vi "Script Rich to Flat Oneof Conversion.vi"(5 "element metadata":T1={"Field Name"="", "Embedded Message Name"="", "Protobuf Index"=1, "MessageElementType"=enum."StringValue", "Repeated"=FALSE, "Is in Oneof"=FALSE, "Oneof Container Name"=""}, 7 "library in":refnum<vi>, 8 "error in (no error)":errorcluster, 9 "unbundler":refnum<vi>, 10 "bundler":refnum<vi>, 11 "vi in":refnum<vi>) -> (0 "error out":errorcluster, 3 "vi out":refnum<vi>)   [LabVIEW 2019, in "gRPC Template Creation Utility.lvlib"]
uses:
  gRPC Template Creation Utility.lvlib
  OneOf Constants/OneOfConstantsEnum.ctl
  TypeDefs/Message Element Type.ctl
  TypeDefs/Message Element Metadata (Scripting).ctl
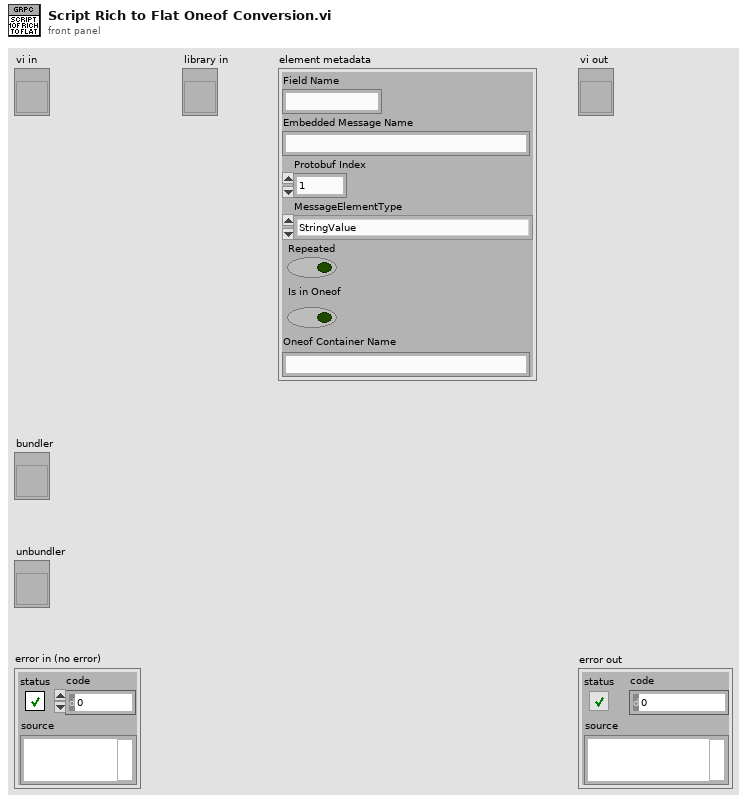
[diagram p1: front panel]
types:
  T1 = typedef "gRPC Template Creation Utility.lvlib/Message Element Metadata (Scripting).ctl" = cluster{"Field Name":string, "Embedded Message Name":string, "Protobuf Index":i32, "MessageElementType":T2, "Repeated":bool, "Is in Oneof":bool, "Oneof Container Name":string}
  T2 = typedef "gRPC Template Creation Utility.lvlib/Message Element Type.ctl" = enum32{"Int32Value", "FloatValue", "DoubleValue", "BoolValue", "StringValue", "MessageValue", "Int64Value", "UInt32Value", "UInt64Value", "EnumValue", "Bytes", "Fixed64", "Fixed32", "SFixed64", "SFixed32", "SInt64", "SInt32"}
  T3 = typedef "gRPC Template Creation Utility.lvlib/OneOfConstantsEnum.ctl" = enum16{"FlatToRichVIPrefix", "RichToFlatVIPrefix", "FlatTypeDefSuffix"}
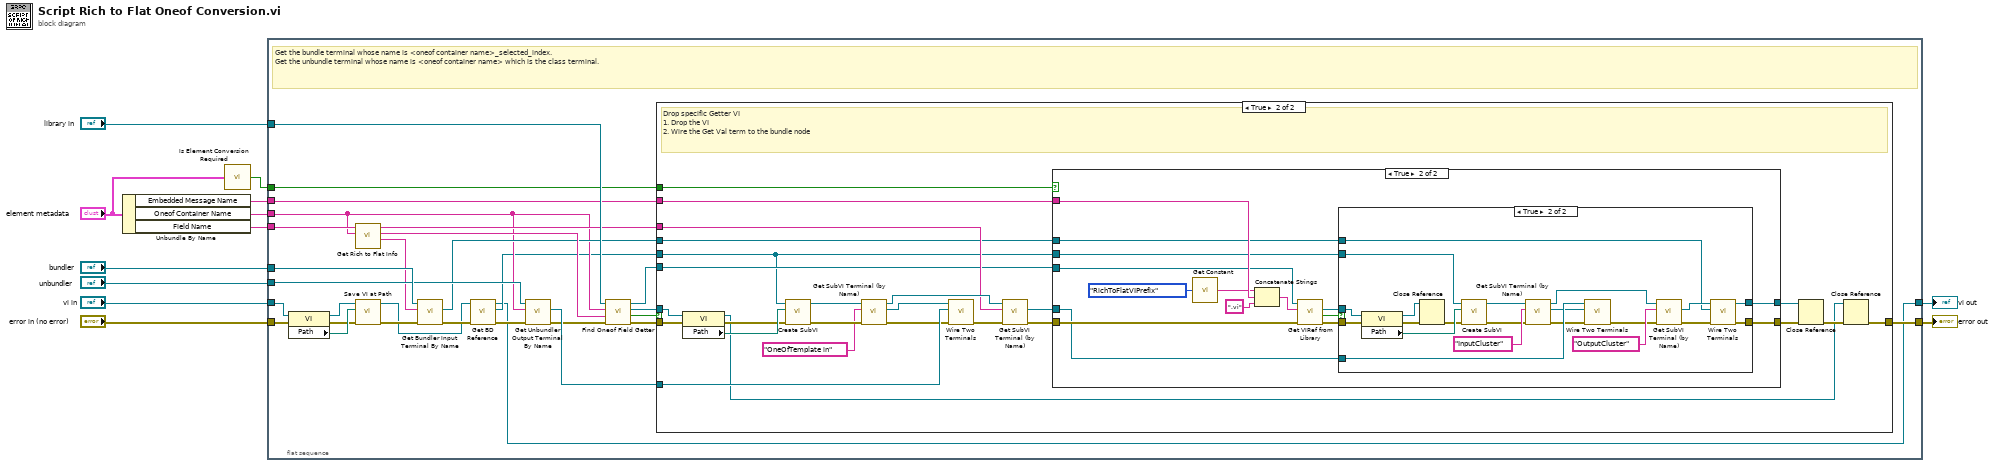
[diagram p0: block diagram]
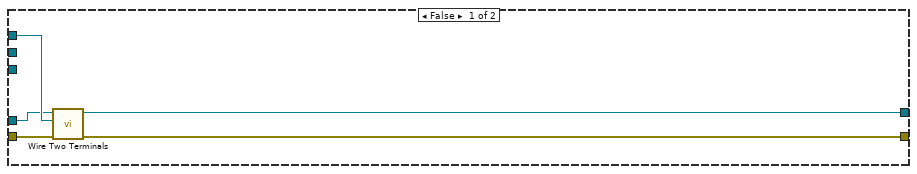
[diagram p3: hidden frame]
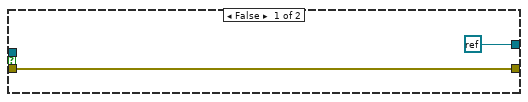
[diagram p4: hidden frame]
diagram:
  n1 = Unbundle By Name("element metadata") -> ("Embedded Message Name"=w7:string, "Oneof Container Name"=w9:string, "Field Name"=w8:string)
  n2 = call "Is Element Conversion Required.vi"("element metadata"="element metadata") -> ("conversion required"=w2:bool)
  n3 = flat-sequence {
    tunnel: w9 -> [w24]
    tunnel: w8 -> [w27]
    tunnel: "error in (no error)" -> [w20]
    tunnel: [w33] -> w11
    tunnel: "bundler" -> [w41]
    tunnel: "unbundler" -> [w40]
    tunnel: "vi in" -> [w39]
    tunnel: "library in" -> [w32]
    tunnel: [w13] -> w12
    tunnel: w2 -> [w23]
    tunnel: w7 -> [w22]
    frame #0 {
      # "Get the bundle terminal whose name is <oneof container name>_selected_index.\nGet the unbundle terminal whose name is <oneof container name> which is the class terminal."
      n4 = property class="VI"(reference=w39, error in=w20) -> (reference out=w31:refnum<vi>, error out=w29:errorcluster, "Path"=w30:path)
      n5 = call "Get Rich to Flat Info.vi"("oneof container name"=w24, "field name"=w27) -> ("bundler terminal name"=w25:string, "getter vi name"=w36:string, "get value terminal name"=w26:string)  [unwired: 7 in]
      n6 = call "Save VI at Path.vi"("error in (no error)"=w29, "Path"=w30, "VI in"=w31) -> ("error out"=w19:errorcluster, "VI out"=w14:refnum<vi>)  [unwired: 6 in, 1 out]
      n7 = call "Get Bundler Input Terminal By Name.vi"("error in (no error)"=w19, "Terminal name"=w25, "Bundler in"=w41) -> ("error out"=w15:errorcluster, "Terminal Refnum"=w28:refnum<vi>)  [unwired: 5 in, 2 out]
      n8 = call "Get BD Reference.vi"("error in"=w15, "VI in"=w14) -> ("error out"=w18:errorcluster, "Block Diagram"=w16:refnum<vi>, "VI out"=w13:refnum<vi>)  [unwired: 7 in]
      n9 = call "Get Unbundler Output Terminal By Name.vi"("error in (no error)"=w18, "Terminal name"=w24, "Unbundler in"=w40) -> ("error out"=w17:errorcluster, "Terminal Refnum"=w35:refnum<vi>)  [unwired: 5 in, 2 out]
      n10 = call "Find Oneof Field Getter.vi"("error in (no error)"=w17, "getter vi name"=w36, "oneof container name"=w24, "library in"=w32) -> ("error out"=w34:errorcluster, "found?"=w37:bool, "getter vi"=w38:refnum<vi>, "library out"=w21:refnum<vi>)  [unwired: 4 in]
      n11 = case shown="True" w37 {
        tunnel: w38 -> [_ w67]
        tunnel: w35 -> [_ w63]
        tunnel: w34 -> [w42 w59]
        tunnel: [w42 w56] -> w33
        tunnel: w28 -> [_ w48]
        tunnel: w16 -> [_ w43]
        tunnel: w26 -> [_ w52]
        tunnel: w23 -> [_ w51]
        tunnel: w22 -> [_ w50]
        tunnel: w21 -> [_ w44]
        frame False {
          # "TODO: Add error because we didn't find the getter VI"
        }
        frame True {
          # "Drop specific Getter VI\n1. Drop the VI\n2. Wire the Get Val term to the bundle node"
          n12 = property class="VI"(reference=w67, error in=w59) -> (reference out=w57:refnum<vi>, error out=w60:errorcluster, "Path"=w66:path)
          n13 = call "Create SubVI.vi"("error in (no error)"=w60, "Path"=w66, "Diagram in"=w43) -> ("error out"=w61:errorcluster, "subVI refnum"=w65:refnum<vi>)  [unwired: 7 in]
          n14 = call "Get SubVI Terminal (by Name).vi"("error in (no error)"=w61, "Terminal name"="OneOfTemplate in", "SubVI in"=w65) -> ("error out"=w62:errorcluster, "SubVI Term ref"=w64:refnum<vi>, "SubVI out"=w54:refnum<vi>)  [unwired: 5 in, 1 out]
          n15 = call "Wire Two Terminals.vi"("error in (no error)"=w62, "Sink Terminal in"=w63, "Source Terminal"=w64) -> ("error out"=w53:errorcluster)  [unwired: 7 in, 1 out]
          n16 = call "Get SubVI Terminal (by Name).vi"("error in (no error)"=w53, "Terminal name"=w52, "SubVI in"=w54) -> ("error out"=w49:errorcluster, "SubVI Term ref"=w47:refnum<vi>)  [unwired: 5 in, 2 out]
          n17 = case shown="True" w51 {
            tunnel: w50 -> [_ w85]
            tunnel: w49 -> [w72 w83]
            tunnel: w48 -> [w71 w76]
            tunnel: w47 -> [w70 w77]
            tunnel: [w69 w78] -> w46
            tunnel: [w68 w75] -> w45
            tunnel: w44 -> [_ w84]
            tunnel: w43 -> [_ w80]
            frame False {
              n18 = call "Wire Two Terminals.vi"("error in (no error)"=w72, "Sink Terminal in"=w71, "Source Terminal"=w70) -> ("error out"=w69:errorcluster, "Source Terminal out"=w68:refnum<vi>)  [unwired: 7 in]
            }
            frame True {
              n19 = call "Get Constant.vi"("Selection"=OneOfConstantsEnum."RichToFlatVIPrefix") -> ("String"=w73:string)
              n20 = Concatenate Strings(w73, w85, ".vi" ("string")) -> (w86:string)
              n21 = call "Get VIRef from Library.vi"("error in (no error)"=w83, "item name"=w86, "library in"=w84) -> ("error out"=w81:errorcluster, "found"=w82:bool, "vi"=w79:refnum<vi>)  [unwired: 5 in, 1 out]
              n22 = case shown="True" w82 {
                tunnel: [w89 w96] -> w78
                tunnel: w81 -> [w89 w94]
                tunnel: w80 -> [_ w110]
                tunnel: w79 -> [_ w109]
                tunnel: w77 -> [_ w104]
                tunnel: w76 -> [_ w93]
                tunnel: [refnum<k0> refnum w95] -> w75
                frame False {
                }
                frame True {
                  n23 = property class="VI"(reference=w109, error in=w94) -> (reference out=w90:refnum<vi>, error out=w92:errorcluster, "Path"=w108:path)
                  n24 = Close Reference(reference=w90, error in (no error)=w92) -> (error out=w91:errorcluster)
                  n25 = call "Create SubVI.vi"("error in (no error)"=w91, "Path"=w108, "Diagram in"=w110) -> ("error out"=w105:errorcluster, "subVI refnum"=w107:refnum<vi>)  [unwired: 7 in]
                  n26 = call "Get SubVI Terminal (by Name).vi"("error in (no error)"=w105, "Terminal name"="InputCluster", "SubVI in"=w107) -> ("error out"=w102:errorcluster, "SubVI Term ref"=w103:refnum<vi>, "SubVI out"=w99:refnum<vi>)  [unwired: 5 in, 1 out]
                  n27 = call "Wire Two Terminals.vi"("error in (no error)"=w102, "Sink Terminal in"=w103, "Source Terminal"=w104) -> ("error out"=w100:errorcluster)  [unwired: 7 in, 1 out]
                  n28 = call "Get SubVI Terminal (by Name).vi"("error in (no error)"=w100, "Terminal name"="OutputCluster", "SubVI in"=w99) -> ("error out"=w97:errorcluster, "SubVI Term ref"=w98:refnum<vi>)  [unwired: 5 in, 2 out]
                  n29 = call "Wire Two Terminals.vi"("error in (no error)"=w97, "Sink Terminal in"=w93, "Source Terminal"=w98) -> ("error out"=w96:errorcluster, "Source Terminal out"=w95:refnum<vi>)  [unwired: 7 in]
                }
              }
            }
          }
          n30 = Close Reference(reference=w45, error in (no error)=w46) -> (error out=w58:errorcluster)
          n31 = Close Reference(reference=w57, error in (no error)=w58) -> (error out=w56:errorcluster)
        }
      }
    }
  }
  "error out" <- w11
  "vi out" <- w12
